vi "InitializeNetworkStreamReader.vi"(11 "Boat Type":T1) -> (0 "error out":errorcluster, 3 "NetworkStreamReader out":refnum<class "NetworkStreamReader.lvclass">)   [LabVIEW 2013]
doc: "Initializes the network stream reader."
uses:
  RIO-OCU_Comm/NetworkStreams/Reader/NetworkStreamReader.lvclass
  cRIO_Code/Data/TypeDefs/BoatType.ctl
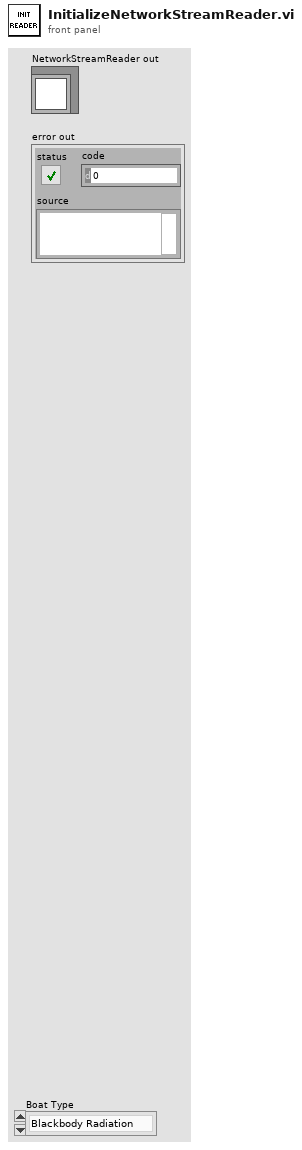
[diagram p1: front panel]
types:
  T1 = typedef "BoatType.ctl" = enum16{"Blackbody Radiation", "ReadLog", "Little boats", "Damn Yankee"}
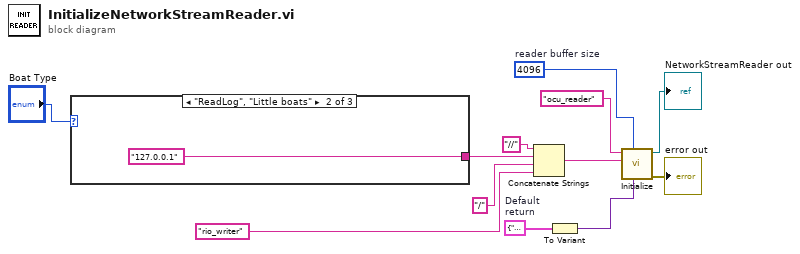
[diagram p0: block diagram]
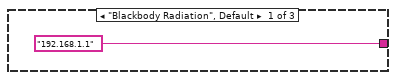
[diagram p2: hidden frame]
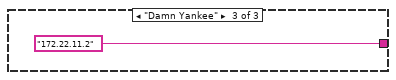
[diagram p3: hidden frame]
diagram:
  w9 = cluster{"Name":string, "value":variant} {"Name"="", "value"=variant}  # Default return
  w6 = 4096  # reader buffer size
  n1 = case shown="\"ReadLog\", \"Little boats\"" "Boat Type" {
    tunnel: ["192.168.1.1" "127.0.0.1" "172.22.11.2"] -> w1
    frame "Blackbody Radiation", Default {
    }
    frame "ReadLog", "Little boats" {
    }
    frame "Damn Yankee" {
    }
  }
  n2 = Concatenate Strings("//" ("string"), w1, "/", "rio_writer" ("string")) -> (w8:string)
  n3 = To Variant(anything=w9) -> (Variant=w10:variant)
  n4 = call "Initialize.vi"("Default return"=w10, "reader buffer size"=w6, "writer url"=w8, "reader name"="ocu_reader" ("writer name")) -> ("error out"=→"error out":errorcluster, "NetworkStreamReader out"=→"NetworkStreamReader out":refnum<class "NetworkStreamReader.lvclass">)  [unwired: 6 in]
